vi "Returning A Value Pointer To Simple Struct Added.vi"(8 "error in (no error)":errorcluster) -> ()   [LabVIEW 2009, in "LabVIEWWrapper_PassingDataSampleDLL.lvlib"]
doc: "int ReturningAValue_Integer (void);"
uses:
  LabVIEWWrapper_PassingDataSampleDLL.lvlib
  CustomControlsForStructs/SimpleStruct Circle.ctl
  PassingDataSampleDLL.dll
panel:
  out "SimpleStruct Circle":T1
  out "error out":errorcluster
  out "Pointer":i64
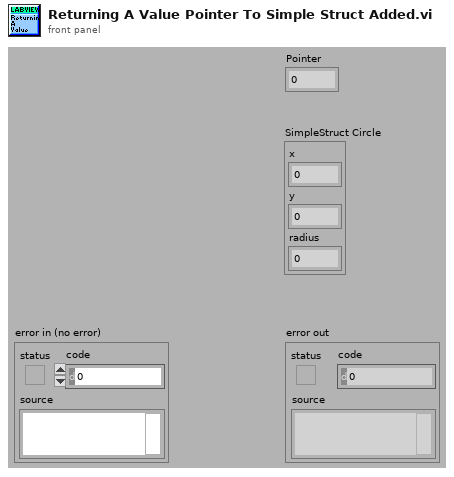
[diagram p1: front panel]
types:
  T1 = typedef "LabVIEWWrapper_PassingDataSampleDLL.lvlib/SimpleStruct Circle.ctl" = cluster{"x":sgl, "y":sgl, "radius":sgl}
  T2 = cluster{"Destination":sgl, "Destination":sgl, "Destination":sgl}
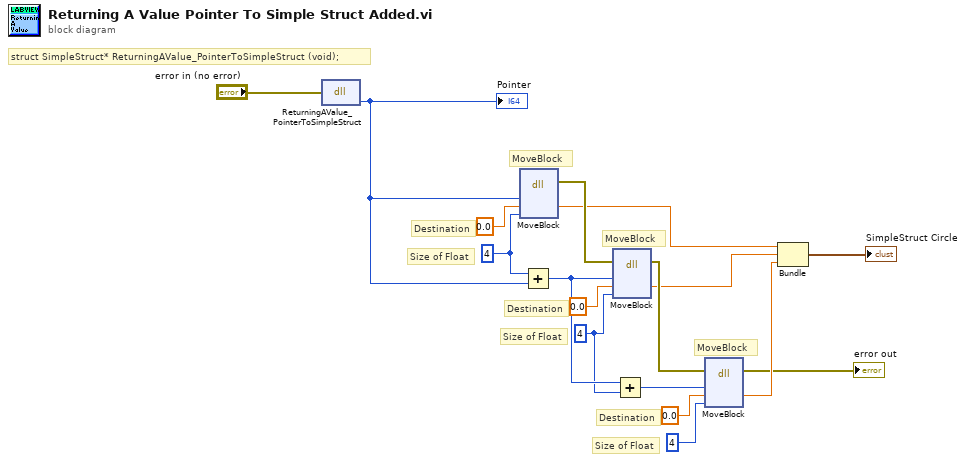
[diagram p0: block diagram]
diagram:
  w7 = 4 ("arg3")
  w12 = 4 ("arg3")
  # "Destination"
  # "Size of Float"
  # "MoveBlock"
  # "Destination"
  # "Size of Float"
  # "MoveBlock"
  # "Destination"
  # "Size of Float"
  # "MoveBlock"
  # "struct SimpleStruct* ReturningAValue_PointerToSimpleStruct (void);"
  n1 = dll-call lib="C:/My Dropbox/Systems Engineering Application/SDK/C Integration/LabVIEWWrapper/PassingDataSampleDLL.*" fn="ReturningAValue_PointerToSimpleStruct"(error in="error in (no error)") -> ("return type"=w13:i64)  [unwired: 2 in, 2 out]
  "Pointer" <- w13
  n2 = dll-call lib="LabVIEW" fn="MoveBlock"("Address (Pointer)"=w13, "Destination"=sgl 0.0, "Size"=w12) -> (error out=w14:errorcluster, "Destination"=w5:sgl)  [unwired: 6 in, 1 out]
  n3 = Add(x=w12, y=w13) -> (x+y=w8:i64)
  n4 = dll-call lib="LabVIEW" fn="MoveBlock"(error in=w14, "Address (Pointer)"=w8, "Destination"=sgl 0.0, "Size"=w7) -> (error out=w6:errorcluster, "Destination"=w4:sgl)  [unwired: 5 in, 1 out]
  n5 = Add(x=w8, y=w7) -> (x+y=w9:i64)
  n6 = dll-call lib="LabVIEW" fn="MoveBlock"(error in=w6, "Address (Pointer)"=w9, "Destination"=sgl 0.0, "Size"=4 ("arg3")) -> (error out=→"error out":errorcluster, "Destination"=w3:sgl)  [unwired: 5 in, 1 out]
  n7 = Bundle("Destination"=w5, "Destination"=w4, "Destination"=w3) -> (→"SimpleStruct Circle":T2)  [unwired: 1 in]
